vi "depth read 2016.vi"(6 "String Pot \nSlope":dbl=1.7339999675750732 format="%.2f", 7 "Sensor Cluster In":T1, 8 "Increment Button":bool, 9 "Read String Pot":bool=TRUE, 10 "Initialize Debug":bool, 11 "Debug":bool) -> (3 "Distance":dbl format="%.2f")   [LabVIEW 2016]
uses:
  Waterloo DAQ/controls/MCC DAQ Readings.ctl
  KPRO_lv2015/ad interface/Global_SIM_switch.vi
  KPRO_lv2015/Kpro Globals.vi
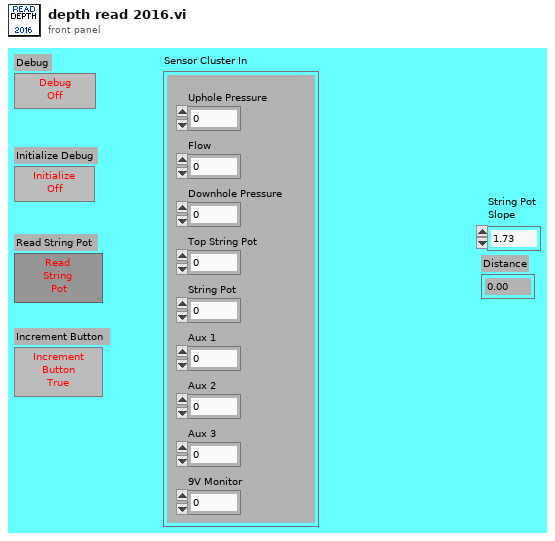
[diagram p1: front panel]
types:
  T1 = typedef "MCC DAQ Readings.ctl" = cluster{"Uphole Pressure":dbl, "Flow":dbl, "Downhole Pressure":dbl, "Top String Pot":dbl, "String Pot":dbl, "Aux 1":dbl, "Aux 2":dbl, "Aux 3":dbl, "9V Monitor":dbl}
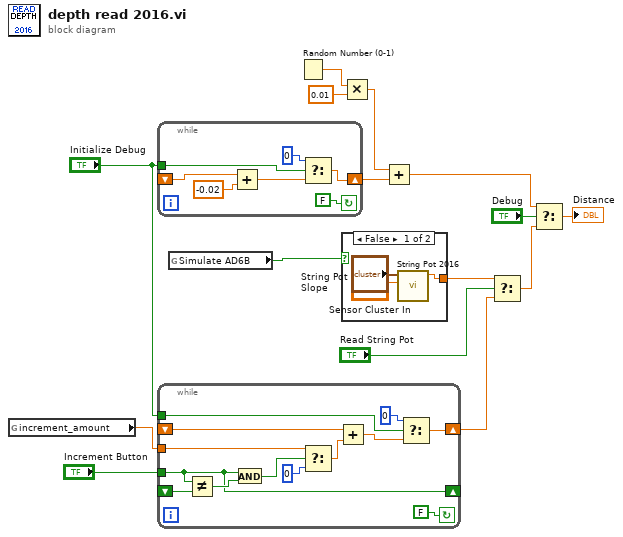
[diagram p0: block diagram]
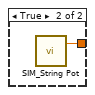
[diagram p2: hidden frame]
diagram:
  n1 = global read "Kpro Globals.vi" "increment_amount"() -> (w1:dbl)
  n2 = while {
    tunnel: "Initialize Debug" -> [w21]
    shift-left: _ -> [w19]
    shift-right: [w20] -> w13
    stop <- FALSE continue-if-true
    n3 = Add(x=w19, y=-0.02) -> (x+y=w17:dbl)
    n4 = Select(t=0, s=w21, f=w17) -> (s? t:f=w20:dbl)
  }
  n5 = while {
    tunnel: w1 -> [w23]
    tunnel: "Increment Button" -> [w25]
    shift-left: _ -> [w30]
    shift-right: [w25] -> _
    tunnel: "Initialize Debug" -> [w31]
    shift-left: _ -> [w33]
    shift-right: [w34] -> w4
    stop <- FALSE continue-if-true
    n6 = Not Equal?(x=w25, y=w30) -> (x != y?=w28:bool)
    n7 = And(x=w25, y=w28) -> (x .and. y?=w26:bool)
    n8 = Select(t=w23, s=w26, f=0) -> (s? t:f=w29:dbl)
    n9 = Add(x=w33, y=w29) -> (x+y=w32:dbl)
    n10 = Select(t=0, s=w31, f=w32) -> (s? t:f=w34:dbl)
  }
  n11 = global read "Global_SIM_switch.vi" "Simulate AD6B"() -> (w2:bool)
  n12 = Random Number (0-1)() -> (number: 0 to 1=w15:dbl)
  n13 = Multiply(x=w15, y=0.01) -> (x*y=w12:dbl)
  n14 = case shown="False" w2 {
    tunnel: [w38 w39] -> w3
    frame False {
      n15 = call "String Pot 2016.vi"("String Pot \nSlope"="String Pot \nSlope", "Sensor Cluster"="Sensor Cluster In") -> ("Distance (in)"=w38:dbl)  [unwired: 9 in]
    }
    frame True {
      n16 = call "SIM_String Pot.vi"() -> ("Distance (in)"=w39:dbl)  [unwired: 3 in]
    }
  }
  n17 = Add(x=w12, y=w13) -> (x+y=w9:dbl)
  n18 = Select(t=w3, s="Read String Pot", f=w4) -> (s? t:f=w8:dbl)
  n19 = Select(t=w9, s="Debug", f=w8) -> (s? t:f=→"Distance":dbl)
